vi "Inst_K2002.vi"(8 "error in":errorcluster, 10 "All Message Queues in":T1, 11 "Prueba31 in":refnum<class "Prueba03.lvclass">) -> (0 "error out":errorcluster)   [LabVIEW 2019, in "Prueba03.lvclass"]
uses:
  Prueba03.lvclass
  QMH/Message Queue/All Message Queues.ctl
  QMH/Message Queue/Message Cluster.ctl
  Prueba03.lvclass/Prueba03.ctl
  <vilib>/Utility/error.llb/Error Cluster From Error Code.vi
  QMH/Message Queue/Enqueue Message (Single).vi
  <vilib>/ErrorRing/Error Ring.xnode
  QMH/Message Queue/Message Queue.lvlib
  Instrumento/Keithley2002/Keithley2002.lvclass
panel:
  out "K_iterac":i32
  out "All States":string[](array[string])
  out "Actual State":string
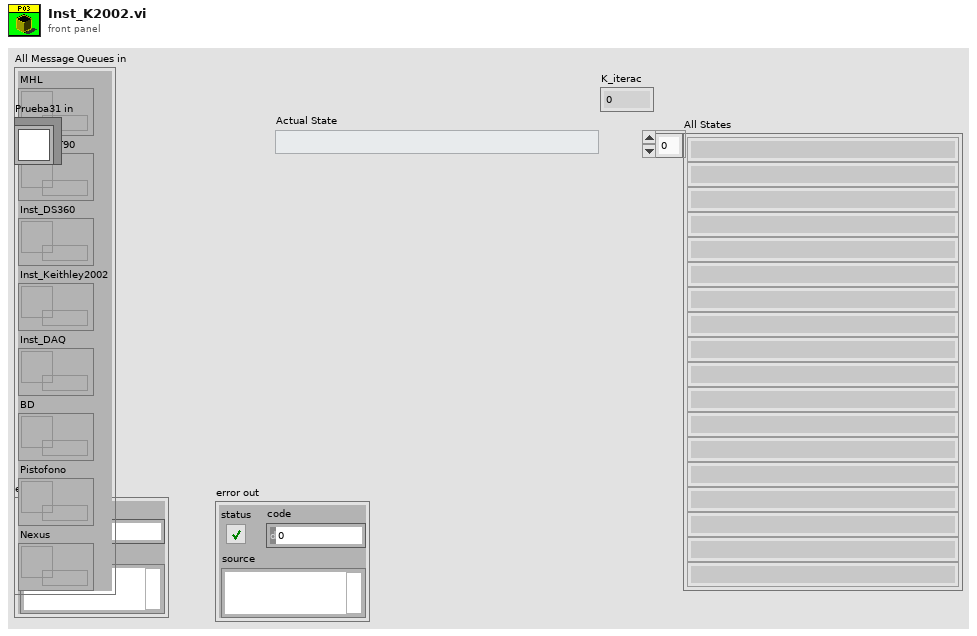
[diagram p1: front panel]
types:
  T1 = typedef "Message Queue.lvlib/All Message Queues.ctl" = cluster{"MHL":refnum<queue>, "Inst_CNT90":refnum<queue>, "Inst_DS360":refnum<queue>, "Inst_Keithley2002":refnum<queue>, "Inst_DAQ":refnum<queue>, "BD":refnum<queue>, "Pistofono":refnum<queue>, "Nexus":refnum<queue>}
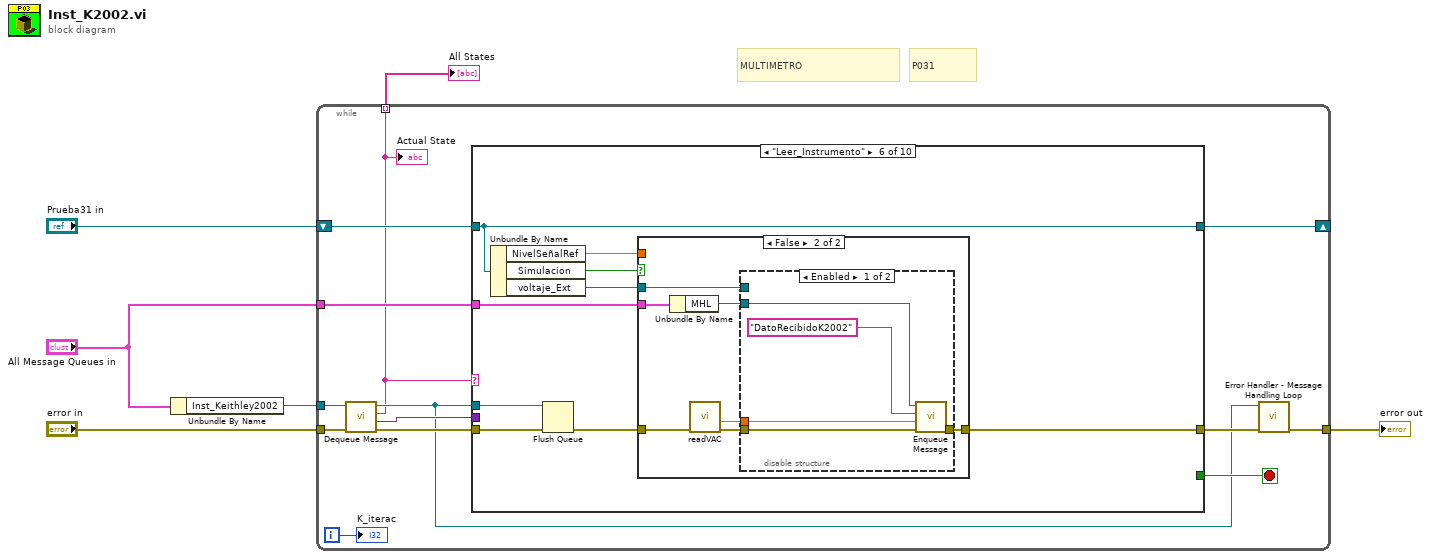
[diagram p0: block diagram]
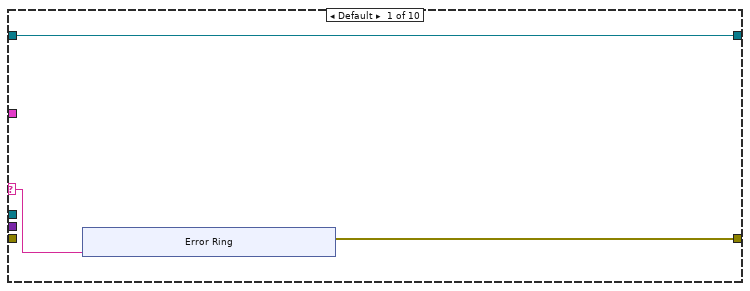
[diagram p2: hidden frame]
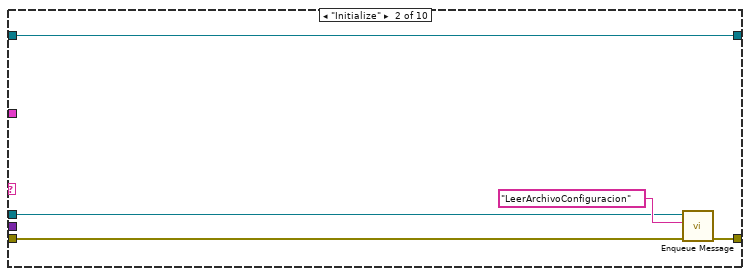
[diagram p3: hidden frame]
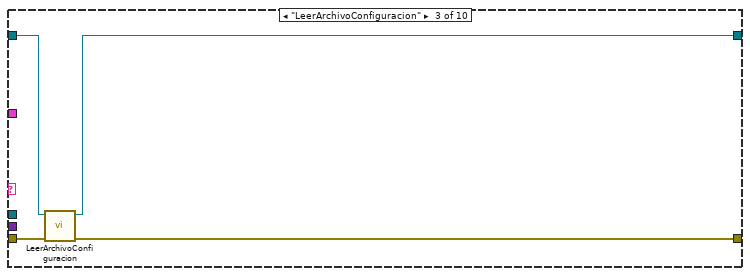
[diagram p4: hidden frame]
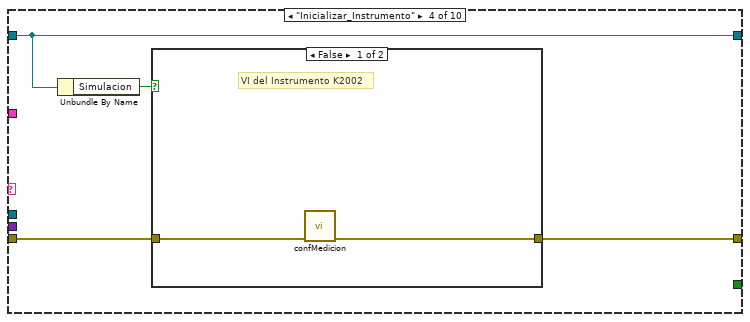
[diagram p5: hidden frame]
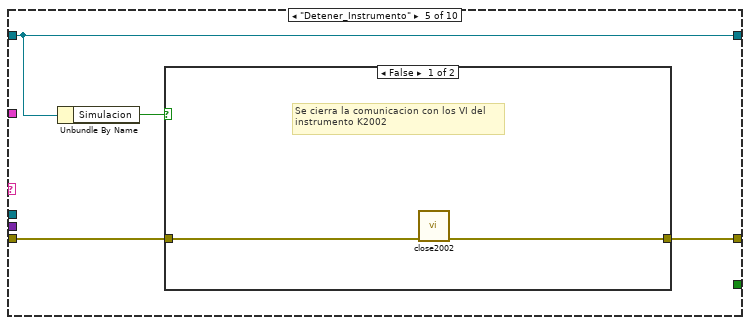
[diagram p7: hidden frame]
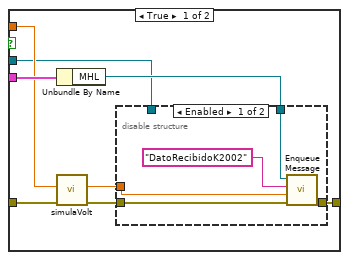
[diagram p9: hidden frame]
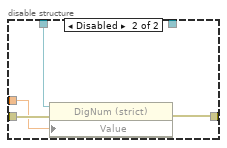
[diagram p10: hidden frame]
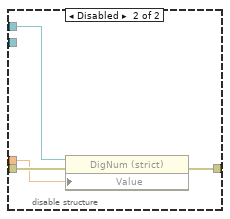
[diagram p11: hidden frame]
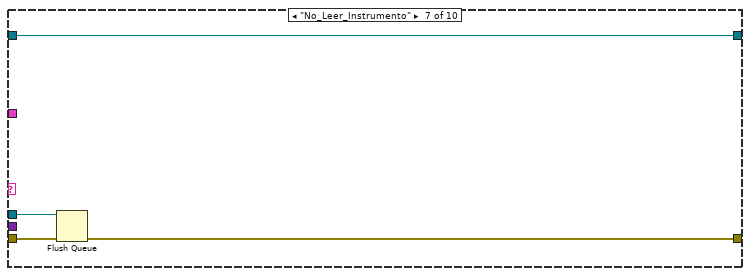
[diagram p12: hidden frame]
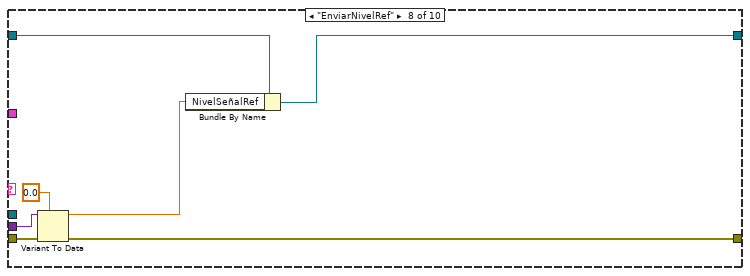
[diagram p13: hidden frame]
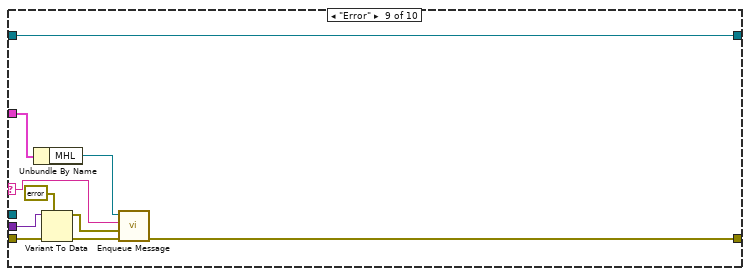
[diagram p14: hidden frame]
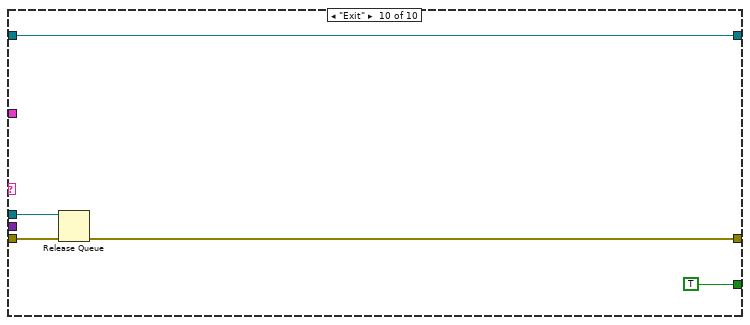
[diagram p15: hidden frame]
diagram:
  # "P031"
  # "MULTIMETRO"
  n1 = Unbundle By Name("All Message Queues in") -> ("Inst_Keithley2002"=w4:refnum<queue>)
  n2 = while {
    tunnel: "error in" -> [w19]
    tunnel: w4 -> [w18]
    tunnel: "All Message Queues in" -> [w17]
    tunnel: [w10] -> w2
    shift-right: [w13] -> _
    shift-left: "Prueba31 in" -> [w16]
    tunnel: [w8] -> w1 mode=indexing
    i -> [w7]
    stop <- w12 stop-if-true
    n3 = call "Dequeue Message.vi"("error in (no error)"=w19, "Message Queue"=w18) -> ("error out"=w14:errorcluster, "Message Data"=w15:variant, "Message"=w8:string, "dup Message Queue"=w9:refnum<queue>)  [unwired: 6 in]
    "Actual State" <- w8
    n4 = case shown="\"Leer_Instrumento\"" w8 {
      selector: w8 -> [w22 _ _ _ _ _ _ _ w108 _]
      tunnel: w17 -> [_ _ _ _ _ w59 _ _ w107 _]
      tunnel: w16 -> [w20 w34 w35 w39 w48 w61 w97 w100 w115 w117]
      tunnel: w9 -> [_ w30 _ _ _ w53 w96 _ _ w119]
      tunnel: w15 -> [_ _ _ _ _ _ _ w102 w112 _]
      tunnel: w14 -> [_ w32 w37 w40 w46 w58 w98 w104 w113 w120]
      tunnel: [w21 w31 w38 w42 w49 w57 w95 w105 w110 w116] -> w11
      tunnel: [w20 w34 w36 w39 w48 w61 w97 w101 w115 w117] -> w13
      tunnel: [_ _ _ _ _ _ _ _ _ TRUE] -> w12
      frame Default {
        n5 = xnode "Error Ring"("parameter 0"=w22) -> ("error out"=w21:errorcluster)
      }
      frame "Initialize" {
        n6 = call-poly "Enqueue Message.vi"("error in (no error)"=w32, "Message"="LeerArchivoConfiguracion", "Message Queue"=w30) -> ("error out"=w31:errorcluster)  [unwired: 7 in, 1 out]
      }
      frame "LeerArchivoConfiguracion" {
        n7 = call "LeerArchivoConfiguracion.vi"("error in"=w37, "Prueba31 in"=w35) -> ("error out"=w38:errorcluster, "Prueba31 out"=w36:refnum<class "Prueba03.lvclass">)  [unwired: 8 in]
      }
      frame "Inicializar_Instrumento" {
        n8 = Unbundle By Name(w39) -> ("Simulacion"=w41:bool)
        n9 = case shown="False" w41 {
          tunnel: [w44 w45] -> w42
          tunnel: w40 -> [w43 w45]
          frame False {
            # "VI del Instrumento K2002"
            n10 = call "confMedicion.vi"("error in (no error)"=w43) -> ("error out"=w44:errorcluster)  [unwired: 9 in, 1 out]
          }
          frame True {
            # "Simulacion"
          }
        }
      }
      frame "Detener_Instrumento" {
        n11 = Unbundle By Name(w48) -> ("Simulacion"=w47:bool)
        n12 = case shown="False" w47 {
          tunnel: [w51 w52] -> w49
          tunnel: w46 -> [w50 w52]
          frame False {
            # "Se cierra la comunicacion con los VI del\ninstrumento K2002"
            n13 = call "close2002.vi"("error in (no error)"=w50) -> ("error out"=w51:errorcluster)  [unwired: 9 in, 1 out]
          }
          frame True {
            # "Simulacion"
          }
        }
      }
      frame "Leer_Instrumento" {
        n14 = Unbundle By Name(w61) -> ("NivelSeñalRef"=w56:dbl, "Simulacion"=w60:bool, "voltaje_Ext"=w55:refnum<vi>)
        n15 = Flush Queue(queue=w53, error in (no error)=w58) -> (error out=w54:errorcluster)  [unwired: 2 out]
        n16 = case shown="False" w60 {
          tunnel: w59 -> [w69 w85]
          tunnel: [w66 w84] -> w57
          tunnel: w54 -> [w68 w82]
          tunnel: w56 -> [w64 _]
          tunnel: w55 -> [w62 w79]
          frame True {
            n17 = Unbundle By Name(w69) -> ("MHL"=w65:refnum<queue>)
            n18 = call "simulaVolt.vi"("error in (no error)"=w68, "volt in"=w64) -> ("error out"=w67:errorcluster, "volt out"=w63:dbl)  [unwired: 7 in, 1 out]
            n19 = disable-structure shown="Enabled" {
              disable-tunnel: w67 -> [w74 w78]
              disable-tunnel: [w73 w77] -> w66
              disable-tunnel: w65 -> [w72 _]
              disable-tunnel: w63 -> [w70 w75]
              disable-tunnel: w62 -> [_ w76]
              frame Enabled {
                n20 = call-poly "Enqueue Message.vi"("error in (no error)"=w74, "Message Data"=w70, "Message"="DatoRecibidoK2002", "Message Queue"=w72) -> ("error out"=w73:errorcluster)  [unwired: 6 in, 1 out]
              }
              frame Disabled {
                n21 = property class="DigNum (strict)"(reference=w76, error in=w78, "Value"=w75) -> (error out=w77:errorcluster)  [unwired: 1 out]
              }
            }
          }
          frame False {
            n22 = Unbundle By Name(w85) -> ("MHL"=w83:refnum<queue>)
            n23 = call "readVAC.vi"("error in (no error)"=w82) -> ("error out"=w81:errorcluster, "medicion"=w80:dbl)  [unwired: 7 in, 2 out]
            n24 = disable-structure shown="Enabled" {
              disable-tunnel: [w90 w93] -> w84
              disable-tunnel: w83 -> [w89 _]
              disable-tunnel: w81 -> [w87 w94]
              disable-tunnel: w80 -> [w86 w91]
              disable-tunnel: w79 -> [_ w92]
              frame Enabled {
                n25 = call-poly "Enqueue Message.vi"("error in (no error)"=w87, "Message Data"=w86, "Message"="DatoRecibidoK2002", "Message Queue"=w89) -> ("error out"=w90:errorcluster)  [unwired: 6 in, 1 out]
              }
              frame Disabled {
                n26 = property class="DigNum (strict)"(reference=w92, error in=w94, "Value"=w91) -> (error out=w93:errorcluster)  [unwired: 1 out]
              }
            }
          }
        }
      }
      frame "No_Leer_Instrumento" {
        n27 = Flush Queue(queue=w96, error in (no error)=w98) -> (error out=w95:errorcluster)  [unwired: 2 out]
      }
      frame "EnviarNivelRef" {
        n28 = Variant To Data(error in=w104, type=0.0, Variant=w102) -> (data=w99:dbl, error out=w105:errorcluster)
        n29 = Bundle By Name(cluster=w100, "NivelSeñalRef"=w99) -> (w101:refnum<class "Prueba03.lvclass">)
      }
      frame "Error" {
        n30 = Unbundle By Name(w107) -> ("MHL"=w106:refnum<queue>)
        n31 = Variant To Data(error in=w113, type=errorcluster {"status"=FALSE, "code"=0, "source"=""} ("error constant"), Variant=w112) -> (data=w109:errorcluster, error out=w111:errorcluster)
        n32 = call-poly "Enqueue Message.vi"("error in (no error)"=w111, "Message Data"=w109, "Message"=w108, "Message Queue"=w106) -> ("error out"=w110:errorcluster)  [unwired: 6 in, 1 out]
      }
      frame "Exit" {
        n33 = Release Queue(queue=w119, error in (no error)=w120) -> (error out=w116:errorcluster)  [unwired: 1 in, 2 out]
      }
    }
    n34 = call "Error Handler - Message Handling Loop.vi"("error in (no error)"=w11, "Message Queue"=w9) -> ("dup error in"=w10:errorcluster)  [unwired: 8 in, 1 out]
    "K_iterac" <- w7
  }
  "error out" <- w2
  "All States" <- w1
